vi "实时小时数据单参数上传.vi"(0 "参数数值":T1={"CODMn"=TRUE, "CODCr"=TRUE, "DO"=TRUE, "铜"=TRUE, "PH"=TRUE, "氨氮"=TRUE, "比电导率"=TRUE, "水温"=TRUE, "盐度(海水)"=TRUE, "浊度"=TRUE, "总氮"=TRUE, "总磷"=TRUE, "叶绿素a"=TRUE, "藻密度"=TRUE, "水位"=TRUE, "流速"=TRUE, "瞬时流量"=TRUE, "累积流量"=TRUE}) -> (4 "数据发送起始时间":timestamp format="%<%.3X\n%Y/%m/%d>T", 6 "实时小时数据上传":bool, 15 "error out":errorcluster)   [LabVIEW 2016, in "数据传输系统.lvlib"]
uses:
  <vilib>/Utility/config.llb/Write Key (String).vi
  <vilib>/Utility/config.llb/NI_LVConfig.lvlib
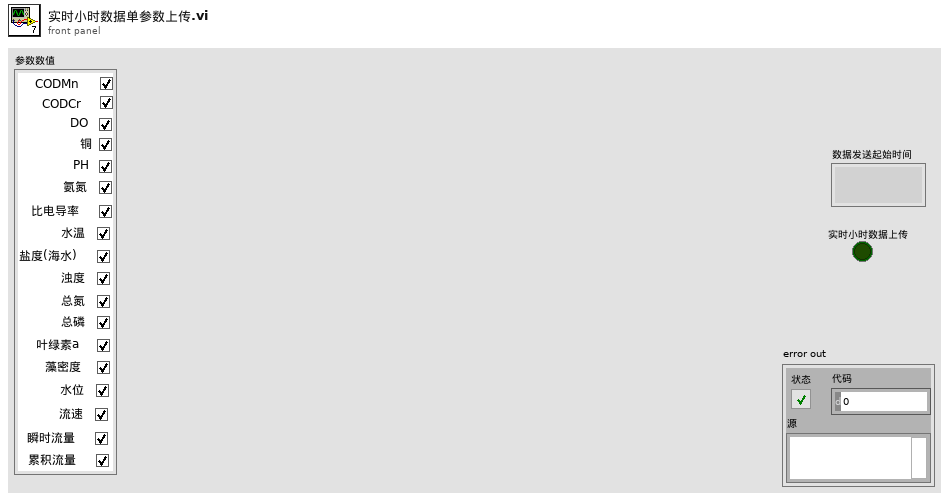
[diagram p1: front panel]
types:
  T1 = cluster{"CODMn":bool, "CODCr":bool, "DO":bool, "铜":bool, "PH":bool, "氨氮":bool, "比电导率":bool, "水温":bool, "盐度(海水)":bool, "浊度":bool, "总氮":bool, "总磷":bool, "叶绿素a":bool, "藻密度":bool, "水位":bool, "流速":bool, "瞬时流量":bool, "累积流量":bool}
  T2 = typedef "NI_LVConfig.lvlib/Config Data RefNum.ctl" = refnum<k1>
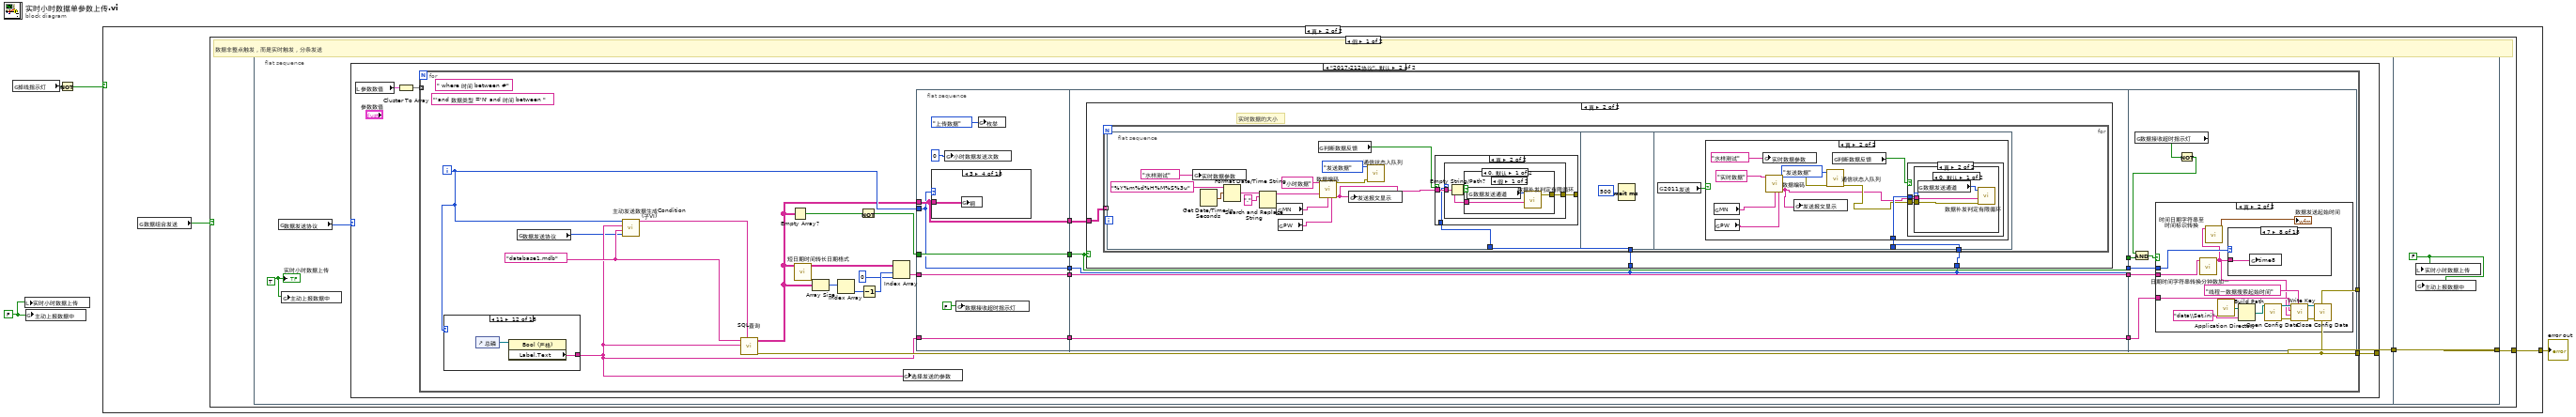
[diagram p0: block diagram]
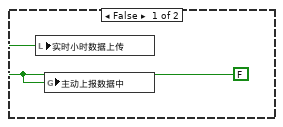
[diagram p2: hidden frame]
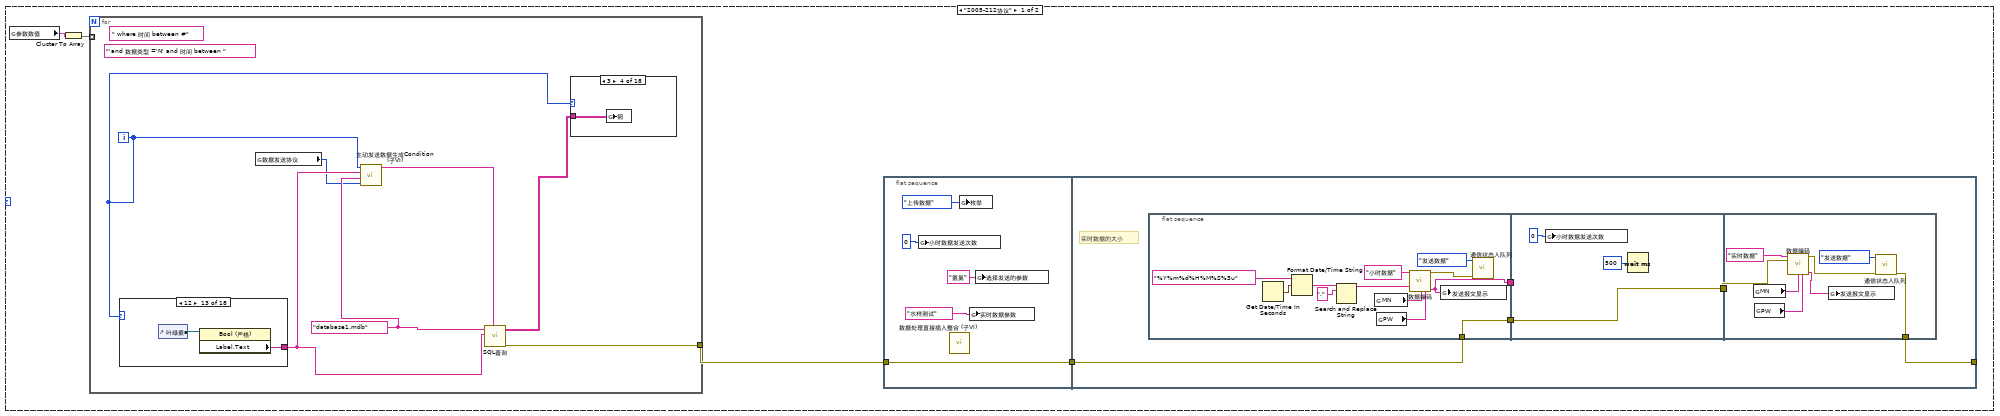
[diagram p3: hidden frame]
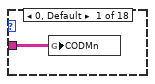
[diagram p4: hidden frame]
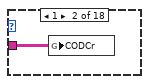
[diagram p5: hidden frame]
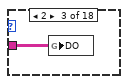
[diagram p6: hidden frame]
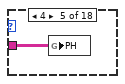
[diagram p7: hidden frame]
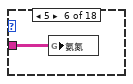
[diagram p8: hidden frame]
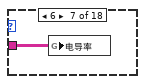
[diagram p9: hidden frame]
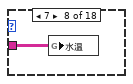
[diagram p10: hidden frame]
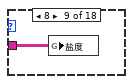
[diagram p11: hidden frame]
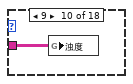
[diagram p12: hidden frame]
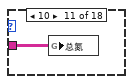
[diagram p13: hidden frame]
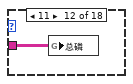
[diagram p14: hidden frame]
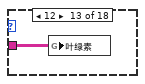
[diagram p15: hidden frame]
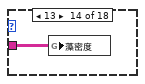
[diagram p16: hidden frame]
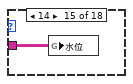
[diagram p17: hidden frame]
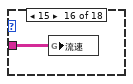
[diagram p18: hidden frame]
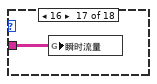
[diagram p19: hidden frame]
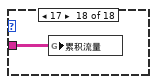
[diagram p20: hidden frame]
diagram:
  w4 = FALSE ("小时数据上传")
  n1 = global read "全局 数据发送重叠.vi" "掉线指示灯"() -> (w3:bool)
  n2 = local write "实时小时数据上传"(w4) -> ()
  n3 = global write "全局 数据发送重叠.vi" "主动上报数据中"(w4) -> ()
  n4 = Not(x=w3) -> (.not. x?=w2:bool)
  n5 = case shown="真" w2 {
    tunnel: [_ w7] -> w1
    frame False {
      w5 = FALSE ("小时数据上传")
      n6 = local write "实时小时数据上传"(w5) -> ()
      n7 = global write "全局 数据发送重叠.vi" "主动上报数据中"(w5) -> ()
    }
    frame True {
      n8 = global read "断电保存全局.vi" "数据组合发送"() -> (w6:bool)
      n9 = case shown="假" w6 {
        tunnel: [w8 _] -> w7
        frame False {
          # "数据非整点触发，而是实时触发，分条发送"
          n10 = flat-sequence {
            tunnel: [w12] -> w9
            tunnel: [w291] -> w8
            tunnel: w9 -> [w291]
            frame #0 {
              w11 = TRUE ("小时数据上传")
              n11 = global read "断电保存全局.vi" "数据发送协议"() -> (w10:enum16{"2005-212协议", "2017-212协议"})
              n12 = global write "全局 数据发送重叠.vi" "主动上报数据中"(w11) -> ()
              n13 = case shown="\"2017-212协议\", 默认" w10 {
                tunnel: [_ w111] -> w12
                frame "2005-212协议" {
                  n14 = global read "全局1.vi" "参数数值"() -> (w13:T1)
                  n15 = Cluster To Array(cluster=w13) -> (array=w16:bool[])
                  n16 = for {
                    tunnel: w16 -> [_] mode=indexing
                    tunnel: [w56] -> w15
                    i -> [w54]
                    (unwired) " where 时间 between #"
                    w52 = "database1.mdb" ("database")
                    (unwired) "'and 数据类型 ='N' and 时间 between "
                    n17 = case shown="12" w54 {
                      tunnel: [w75 w77 w79 w81 w83 w85 w87 w89 w91 w93 w95 w97 w99 w101 w103 w105 w107 w109] -> w53
                      frame 0, Default {
                        n18 = control-ref of="CODMn"() -> (w76:refnum<vi>)
                        n19 = property class="Bool (严格)"(reference=w76) -> ("Label.Text"=w75:string)  [unwired: 1 in, 2 out]
                      }
                      frame 1 {
                        n20 = control-ref of="CODCr"() -> (w78:refnum<vi>)
                        n21 = property class="Bool (严格)"(reference=w78) -> ("Label.Text"=w77:string)  [unwired: 1 in, 2 out]
                      }
                      frame 2 {
                        n22 = control-ref of="DO"() -> (w80:refnum<vi>)
                        n23 = property class="Bool (严格)"(reference=w80) -> ("Label.Text"=w79:string)  [unwired: 1 in, 2 out]
                      }
                      frame 3 {
                        n24 = control-ref of="铜"() -> (w82:refnum<vi>)
                        n25 = property class="Bool (严格)"(reference=w82) -> ("Label.Text"=w81:string)  [unwired: 1 in, 2 out]
                      }
                      frame 4 {
                        n26 = control-ref of="PH"() -> (w84:refnum<vi>)
                        n27 = property class="Bool (严格)"(reference=w84) -> ("Label.Text"=w83:string)  [unwired: 1 in, 2 out]
                      }
                      frame 5 {
                        n28 = control-ref of="氨氮"() -> (w86:refnum<vi>)
                        n29 = property class="Bool (严格)"(reference=w86) -> ("Label.Text"=w85:string)  [unwired: 1 in, 2 out]
                      }
                      frame 6 {
                        n30 = control-ref of="比电导率"() -> (w88:refnum<vi>)
                        n31 = property class="Bool (严格)"(reference=w88) -> ("Label.Text"=w87:string)  [unwired: 1 in, 2 out]
                      }
                      frame 7 {
                        n32 = control-ref of="水温"() -> (w90:refnum<vi>)
                        n33 = property class="Bool (严格)"(reference=w90) -> ("Label.Text"=w89:string)  [unwired: 1 in, 2 out]
                      }
                      frame 8 {
                        n34 = control-ref of="盐度(海水)"() -> (w92:refnum<vi>)
                        n35 = property class="Bool (严格)"(reference=w92) -> ("Label.Text"=w91:string)  [unwired: 1 in, 2 out]
                      }
                      frame 9 {
                        n36 = control-ref of="浊度"() -> (w94:refnum<vi>)
                        n37 = property class="Bool (严格)"(reference=w94) -> ("Label.Text"=w93:string)  [unwired: 1 in, 2 out]
                      }
                      frame 10 {
                        n38 = control-ref of="总氮"() -> (w96:refnum<vi>)
                        n39 = property class="Bool (严格)"(reference=w96) -> ("Label.Text"=w95:string)  [unwired: 1 in, 2 out]
                      }
                      frame 11 {
                        n40 = control-ref of="总磷"() -> (w98:refnum<vi>)
                        n41 = property class="Bool (严格)"(reference=w98) -> ("Label.Text"=w97:string)  [unwired: 1 in, 2 out]
                      }
                      frame 12 {
                        n42 = control-ref of="叶绿素a"() -> (w100:refnum<vi>)
                        n43 = property class="Bool (严格)"(reference=w100) -> ("Label.Text"=w99:string)  [unwired: 1 in, 2 out]
                      }
                      frame 13 {
                        n44 = control-ref of="藻密度"() -> (w102:refnum<vi>)
                        n45 = property class="Bool (严格)"(reference=w102) -> ("Label.Text"=w101:string)  [unwired: 1 in, 2 out]
                      }
                      frame 14 {
                        n46 = control-ref of="水位"() -> (w104:refnum<vi>)
                        n47 = property class="Bool (严格)"(reference=w104) -> ("Label.Text"=w103:string)  [unwired: 1 in, 2 out]
                      }
                      frame 15 {
                        n48 = control-ref of="流速"() -> (w106:refnum<vi>)
                        n49 = property class="Bool (严格)"(reference=w106) -> ("Label.Text"=w105:string)  [unwired: 1 in, 2 out]
                      }
                      frame 16 {
                        n50 = control-ref of="瞬时流量"() -> (w108:refnum<vi>)
                        n51 = property class="Bool (严格)"(reference=w108) -> ("Label.Text"=w107:string)  [unwired: 1 in, 2 out]
                      }
                      frame 17 {
                        n52 = control-ref of="累积流量"() -> (w110:refnum<vi>)
                        n53 = property class="Bool (严格)"(reference=w110) -> ("Label.Text"=w109:string)  [unwired: 1 in, 2 out]
                      }
                    }
                    n54 = global read "断电保存全局.vi" "数据发送协议"() -> (w50:enum16{"2005-212协议", "2017-212协议"})
                    n55 = call "主动发送数据生成Condition(子VI).vi"("数据发送协议"=w50, "database"=w52, "Label.Text"=w53, "数值"=w54) -> ("CONDITION"=w51:string)  [unwired: 7 in]
                    n56 = call "SQL查询.vi"("condition"=w51, "table输入"=w53, "database"=w52) -> ("error out"=w56:errorcluster, "data"=w55:string[][])  [unwired: 7 in]
                    n57 = case shown="3" w54 {
                      tunnel: w55 -> [w57 w58 w59 w60 w61 w62 w63 w64 w65 w66 w67 w68 w69 w70 w71 w72 w73 w74]
                      frame 0, Default {
                        n58 = global write "全局 所有参数.vi" "CODMn"(w57) -> ()
                      }
                      frame 1 {
                        n59 = global write "全局 所有参数.vi" "CODCr"(w58) -> ()
                      }
                      frame 2 {
                        n60 = global write "全局 所有参数.vi" "DO"(w59) -> ()
                      }
                      frame 3 {
                        n61 = global write "全局 所有参数.vi" "铜"(w60) -> ()
                      }
                      frame 4 {
                        n62 = global write "全局 所有参数.vi" "PH"(w61) -> ()
                      }
                      frame 5 {
                        n63 = global write "全局 所有参数.vi" "氨氮"(w62) -> ()
                      }
                      frame 6 {
                        n64 = global write "全局 所有参数.vi" "电导率"(w63) -> ()
                      }
                      frame 7 {
                        n65 = global write "全局 所有参数.vi" "水温"(w64) -> ()
                      }
                      frame 8 {
                        n66 = global write "全局 所有参数.vi" "盐度"(w65) -> ()
                      }
                      frame 9 {
                        n67 = global write "全局 所有参数.vi" "浊度"(w66) -> ()
                      }
                      frame 10 {
                        n68 = global write "全局 所有参数.vi" "总氮"(w67) -> ()
                      }
                      frame 11 {
                        n69 = global write "全局 所有参数.vi" "总磷"(w68) -> ()
                      }
                      frame 12 {
                        n70 = global write "全局 所有参数.vi" "叶绿素"(w69) -> ()
                      }
                      frame 13 {
                        n71 = global write "全局 所有参数.vi" "藻密度"(w70) -> ()
                      }
                      frame 14 {
                        n72 = global write "全局 所有参数.vi" "水位"(w71) -> ()
                      }
                      frame 15 {
                        n73 = global write "全局 所有参数.vi" "流速"(w72) -> ()
                      }
                      frame 16 {
                        n74 = global write "全局 所有参数.vi" "瞬时流量"(w73) -> ()
                      }
                      frame 17 {
                        n75 = global write "全局 所有参数.vi" "累积流量"(w74) -> ()
                      }
                    }
                  }
                  n76 = flat-sequence {
                    tunnel: w15 -> [w17]
                    tunnel: [w17] -> w14
                    tunnel: w14 -> [w23]
                    tunnel: [w22] -> _
                    frame #0 {
                      n77 = global write "全局 小时数据发送次数.vi" "小时数据发送次数"(0 ("小时数据发送次数")) -> ()
                      n78 = call "数据处理直接插入整合 (子VI).vi"() -> ()  [unwired: 12 in]
                      n79 = global write "全局1.vi" "枚举"(enum16{"返回请求应答", "上传数据", "返回执行结果"}."上传数据" ("枚举")) -> ()
                      n80 = global write "全局 实时数据参数.vi" "实时数据参数"("水样测试" ("实时数据参数")) -> ()
                      n81 = global write "全局 水样时间.vi" "选择发送的参数"("氨氮" ("选择发送的参数")) -> ()
                    }
                    frame #1 {
                      # "实时数据的大小"
                      n82 = flat-sequence {
                        tunnel: [w32] -> w26
                        tunnel: [w27] -> w24
                        tunnel: w23 -> [w27]
                        tunnel: w26 -> [_]
                        tunnel: [w40] -> w25
                        tunnel: w24 -> [w40]
                        tunnel: w25 -> [w48]
                        tunnel: [w42] -> w22
                        frame #0 {
                          n83 = Get Date/Time In Seconds() -> (seconds since 1Jan1904=w35:timestamp)
                          n84 = Format Date/Time String(time format string (%c)="%Y%m%d%H%M%S%3u" ("时间格式字符串(%c)"), seconds (now)=w35) -> (date/time string=w36:string)  [unwired: 1 in]
                          n85 = Search and Replace String(input string=w36, search string="." ("搜索字符串")) -> (result string=w38:string)  [unwired: 6 in, 3 out]
                          n86 = global read "断电保存全局.vi" "MN"() -> (w30:string)
                          n87 = global read "断电保存全局.vi" "PW"() -> (w29:string)
                          n88 = call "数据编码.vi"("table输入"="小时数据" ("新元素/子数组"), "QN"=w38, "MN"=w30, "PW"=w29) -> ("错误常量"=w28:errorcluster, "通讯包字符串"=w32:string)  [unwired: 10 in]
                          n89 = global write "全局1.vi" "发送报文显示"(w32) -> ()
                          n90 = call "通信状态入队列.vi"("错误输入（无错误）"=w28, "枚举"=enum16{"打开连接", "发送数据", "读取数据", "数据处理", "关闭连接"}."发送数据") -> ()  [unwired: 9 in, 1 out]
                        }
                        frame #1 {
                          n91 = global write "全局 小时数据发送次数.vi" "小时数据发送次数"(0 ("小时数据发送次数")) -> ()
                          n92 = Wait (ms)(milliseconds to wait=u32 500 ("等待时间（毫秒）")) -> ()  [unwired: 1 out]
                        }
                        frame #2 {
                          n93 = global read "断电保存全局.vi" "MN"() -> (w44:string)
                          n94 = global read "断电保存全局.vi" "PW"() -> (w45:string)
                          n95 = call "数据编码.vi"("table输入"="实时数据" ("新元素/子数组"), "错误常量 2"=w48, "MN"=w44, "PW"=w45) -> ("错误常量"=w43:errorcluster, "通讯包字符串"=w47:string)  [unwired: 10 in]
                          n96 = global write "全局1.vi" "发送报文显示"(w47) -> ()
                          n97 = call "通信状态入队列.vi"("错误输入（无错误）"=w43, "枚举"=enum16{"打开连接", "发送数据", "读取数据", "数据处理", "关闭连接"}."发送数据") -> ("错误输出"=w42:errorcluster)  [unwired: 9 in]
                        }
                      }
                    }
                  }
                }
                frame "2017-212协议", Default {
                  n98 = local read "参数数值"() -> (w113:T1)
                  n99 = Cluster To Array(cluster=w113) -> (array=w112:bool[])
                  n100 = for {
                    tunnel: w112 -> [_] mode=indexing
                    tunnel: [w123] -> w111
                    tunnel: [w123] -> _
                    i -> [w122]
                    (unwired) " where 时间 between #"
                    w121 = "database1.mdb" ("database")
                    (unwired) "'and 数据类型 ='N' and 时间 between "
                    n101 = case shown="11" w122 {
                      tunnel: [w254 w256 w258 w260 w262 w264 w266 w268 w270 w272 w274 w276 w278 w280 w282 w284 w286 w288] -> w120
                      frame 0, Default {
                        n102 = control-ref of="CODMn"() -> (w255:refnum<vi>)
                        n103 = property class="Bool (严格)"(reference=w255) -> ("Label.Text"=w254:string)  [unwired: 1 in, 2 out]
                      }
                      frame 1 {
                        n104 = control-ref of="CODCr"() -> (w257:refnum<vi>)
                        n105 = property class="Bool (严格)"(reference=w257) -> ("Label.Text"=w256:string)  [unwired: 1 in, 2 out]
                      }
                      frame 2 {
                        n106 = control-ref of="DO"() -> (w259:refnum<vi>)
                        n107 = property class="Bool (严格)"(reference=w259) -> ("Label.Text"=w258:string)  [unwired: 1 in, 2 out]
                      }
                      frame 3 {
                        n108 = control-ref of="铜"() -> (w261:refnum<vi>)
                        n109 = property class="Bool (严格)"(reference=w261) -> ("Label.Text"=w260:string)  [unwired: 1 in, 2 out]
                      }
                      frame 4 {
                        n110 = control-ref of="PH"() -> (w263:refnum<vi>)
                        n111 = property class="Bool (严格)"(reference=w263) -> ("Label.Text"=w262:string)  [unwired: 1 in, 2 out]
                      }
                      frame 5 {
                        n112 = control-ref of="氨氮"() -> (w265:refnum<vi>)
                        n113 = property class="Bool (严格)"(reference=w265) -> ("Label.Text"=w264:string)  [unwired: 1 in, 2 out]
                      }
                      frame 6 {
                        n114 = control-ref of="比电导率"() -> (w267:refnum<vi>)
                        n115 = property class="Bool (严格)"(reference=w267) -> ("Label.Text"=w266:string)  [unwired: 1 in, 2 out]
                      }
                      frame 7 {
                        n116 = control-ref of="水温"() -> (w269:refnum<vi>)
                        n117 = property class="Bool (严格)"(reference=w269) -> ("Label.Text"=w268:string)  [unwired: 1 in, 2 out]
                      }
                      frame 8 {
                        n118 = control-ref of="盐度(海水)"() -> (w271:refnum<vi>)
                        n119 = property class="Bool (严格)"(reference=w271) -> ("Label.Text"=w270:string)  [unwired: 1 in, 2 out]
                      }
                      frame 9 {
                        n120 = control-ref of="浊度"() -> (w273:refnum<vi>)
                        n121 = property class="Bool (严格)"(reference=w273) -> ("Label.Text"=w272:string)  [unwired: 1 in, 2 out]
                      }
                      frame 10 {
                        n122 = control-ref of="总氮"() -> (w275:refnum<vi>)
                        n123 = property class="Bool (严格)"(reference=w275) -> ("Label.Text"=w274:string)  [unwired: 1 in, 2 out]
                      }
                      frame 11 {
                        n124 = control-ref of="总磷"() -> (w277:refnum<vi>)
                        n125 = property class="Bool (严格)"(reference=w277) -> ("Label.Text"=w276:string)  [unwired: 1 in, 2 out]
                      }
                      frame 12 {
                        n126 = control-ref of="叶绿素a"() -> (w279:refnum<vi>)
                        n127 = property class="Bool (严格)"(reference=w279) -> ("Label.Text"=w278:string)  [unwired: 1 in, 2 out]
                      }
                      frame 13 {
                        n128 = control-ref of="藻密度"() -> (w281:refnum<vi>)
                        n129 = property class="Bool (严格)"(reference=w281) -> ("Label.Text"=w280:string)  [unwired: 1 in, 2 out]
                      }
                      frame 14 {
                        n130 = control-ref of="水位"() -> (w283:refnum<vi>)
                        n131 = property class="Bool (严格)"(reference=w283) -> ("Label.Text"=w282:string)  [unwired: 1 in, 2 out]
                      }
                      frame 15 {
                        n132 = control-ref of="流速"() -> (w285:refnum<vi>)
                        n133 = property class="Bool (严格)"(reference=w285) -> ("Label.Text"=w284:string)  [unwired: 1 in, 2 out]
                      }
                      frame 16 {
                        n134 = control-ref of="瞬时流量"() -> (w287:refnum<vi>)
                        n135 = property class="Bool (严格)"(reference=w287) -> ("Label.Text"=w286:string)  [unwired: 1 in, 2 out]
                      }
                      frame 17 {
                        n136 = control-ref of="累积流量"() -> (w289:refnum<vi>)
                        n137 = property class="Bool (严格)"(reference=w289) -> ("Label.Text"=w288:string)  [unwired: 1 in, 2 out]
                      }
                    }
                    n138 = global read "断电保存全局.vi" "数据发送协议"() -> (w119:enum16{"2005-212协议", "2017-212协议"})
                    n139 = call "主动发送数据生成Condition(子VI).vi"("数据发送协议"=w119, "database"=w121, "Label.Text"=w120, "数值"=w122) -> ("CONDITION"=w137:string)  [unwired: 7 in]
                    n140 = call "SQL查询.vi"("condition"=w137, "table输入"=w120, "database"=w121) -> ("error out"=w123:errorcluster, "data"=w116:string[][])  [unwired: 7 in]
                    n141 = Empty Array?(array=w116) -> (empty?=w136:bool)
                    n142 = call "短日期时间转长日期格式.vi"("data"=w116) -> ("输出数组"=w135:string[][])  [unwired: 10 in]
                    n143 = Array Size(array=w116) -> (size(s)=w118:i32[])
                    n144 = Index Array(array=w118) -> (element=w117:i32)  [unwired: 1 in]
                    n145 = Not(x=w136) -> (.not. x?=w132:bool)
                    n146 = Decrement(x=w117) -> (x-1=w115:i32)
                    n147 = Index Array(array=w135, index (row)=w115, index (col)=0 ("禁用的索引 (列)")) -> (element=w129:string)
                    n148 = global write "全局 水样时间.vi" "选择发送的参数"(w120) -> ()
                    n149 = flat-sequence {
                      tunnel: [w145] -> w134
                      tunnel: [w144] -> w133
                      tunnel: w132 -> [w145]
                      tunnel: w116 -> [w144]
                      tunnel: w122 -> [w139]
                      tunnel: w120 -> [w141]
                      tunnel: [w141] -> w130
                      tunnel: w129 -> [w140]
                      tunnel: [w140] -> w127
                      tunnel: [w139] -> w124
                      tunnel: w134 -> [w165]
                      tunnel: w133 -> [w168]
                      tunnel: [w167] -> w131
                      tunnel: w130 -> [w167]
                      tunnel: [w166] -> w128
                      tunnel: w127 -> [w166]
                      tunnel: [w165] -> w126
                      tunnel: [w164] -> w125
                      tunnel: w124 -> [w164]
                      tunnel: w131 -> [w222]
                      tunnel: w128 -> [w221]
                      tunnel: w126 -> [w219]
                      tunnel: w125 -> [w220]
                      frame #0 {
                        n150 = case shown="3" w139 {
                          tunnel: w144 -> [w146 w147 w148 w149 w150 w151 w152 w153 w154 w155 w156 w157 w158 w159 w160 w161 w162 w163]
                          frame 0, Default {
                            n151 = global write "全局 所有参数.vi" "CODMn"(w146) -> ()
                          }
                          frame 1 {
                            n152 = global write "全局 所有参数.vi" "CODCr"(w147) -> ()
                          }
                          frame 2 {
                            n153 = global write "全局 所有参数.vi" "DO"(w148) -> ()
                          }
                          frame 3 {
                            n154 = global write "全局 所有参数.vi" "铜"(w149) -> ()
                          }
                          frame 4 {
                            n155 = global write "全局 所有参数.vi" "PH"(w150) -> ()
                          }
                          frame 5 {
                            n156 = global write "全局 所有参数.vi" "氨氮"(w151) -> ()
                          }
                          frame 6 {
                            n157 = global write "全局 所有参数.vi" "电导率"(w152) -> ()
                          }
                          frame 7 {
                            n158 = global write "全局 所有参数.vi" "水温"(w153) -> ()
                          }
                          frame 8 {
                            n159 = global write "全局 所有参数.vi" "盐度"(w154) -> ()
                          }
                          frame 9 {
                            n160 = global write "全局 所有参数.vi" "浊度"(w155) -> ()
                          }
                          frame 10 {
                            n161 = global write "全局 所有参数.vi" "总氮"(w156) -> ()
                          }
                          frame 11 {
                            n162 = global write "全局 所有参数.vi" "总磷"(w157) -> ()
                          }
                          frame 12 {
                            n163 = global write "全局 所有参数.vi" "叶绿素"(w158) -> ()
                          }
                          frame 13 {
                            n164 = global write "全局 所有参数.vi" "藻密度"(w159) -> ()
                          }
                          frame 14 {
                            n165 = global write "全局 所有参数.vi" "水位"(w160) -> ()
                          }
                          frame 15 {
                            n166 = global write "全局 所有参数.vi" "流速"(w161) -> ()
                          }
                          frame 16 {
                            n167 = global write "全局 所有参数.vi" "瞬时流量"(w162) -> ()
                          }
                          frame 17 {
                            n168 = global write "全局 所有参数.vi" "累积流量"(w163) -> ()
                          }
                        }
                        n169 = global write "全局 小时数据发送次数.vi" "小时数据发送次数"(0 ("小时数据发送次数")) -> ()
                        n170 = global write "全局 数据发送重叠.vi" "数据接收超时指示灯"(FALSE ("数据接收超时指示灯")) -> ()
                        n171 = global write "全局1.vi" "枚举"(enum16{"返回请求应答", "上传数据", "返回执行结果"}."上传数据" ("枚举")) -> ()
                      }
                      frame #1 {
                        n172 = case shown="真" w165 {
                          tunnel: w168 -> [_ w171]
                          tunnel: w164 -> [_ w170]
                          tunnel: w164 -> [_ w169]
                          frame False {
                          }
                          frame True {
                            # "实时数据的大小"
                            n173 = for {
                              tunnel: w171 -> [_] mode=indexing
                              tunnel: w170 -> [w173]
                              tunnel: w169 -> [w172]
                              n174 = flat-sequence {
                                tunnel: w173 -> [w187]
                                tunnel: w172 -> [w198]
                                frame #0 {
                                n175 = global write "全局 实时数据参数.vi" "实时数据参数"("水样测试" ("实时数据参数")) -> ()
                                n176 = Get Date/Time In Seconds() -> (seconds since 1Jan1904=w183:timestamp)
                                n177 = Format Date/Time String(time format string (%c)="%Y%m%d%H%M%S%3u" ("时间格式字符串(%c)"), seconds (now)=w183) -> (date/time string=w184:string)  [unwired: 1 in]
                                n178 = Search and Replace String(input string=w184, search string="." ("搜索字符串")) -> (result string=w186:string)  [unwired: 6 in, 3 out]
                                n179 = global read "断电保存全局.vi" "MN"() -> (w179:string)
                                n180 = global read "断电保存全局.vi" "PW"() -> (w178:string)
                                n181 = global read "断电保存全局.vi" "判断数据反馈"() -> (w175:bool)
                                n182 = call "数据编码.vi"("table输入"="小时数据" ("新元素/子数组"), "QN"=w186, "MN"=w179, "PW"=w178) -> ("错误常量"=w176:errorcluster, "通讯包字符串"=w174:string)  [unwired: 10 in]
                                n183 = global write "全局1.vi" "发送报文显示"(w174) -> ()
                                n184 = call "通信状态入队列.vi"("错误输入（无错误）"=w176, "枚举"=enum16{"打开连接", "发送数据", "读取数据", "数据处理", "关闭连接"}."发送数据") -> ()  [unwired: 9 in, 1 out]
                                n185 = case shown="真" w175 {
                                tunnel: [_ w190] -> _
                                tunnel: w174 -> [_ w189]
                                tunnel: w187 -> [_ w188]
                                frame False {
                                }
                                frame True {
                                n186 = case shown="0, 默认" w188 {
                                tunnel: [w192 _] -> w190
                                tunnel: w189 -> [w191 _]
                                frame 0, Default {
                                n187 = Empty String/Path?(string/path=w191) -> (empty?=w193:bool)
                                n188 = case shown="假" w193 {
                                tunnel: [w196 _] -> w192
                                tunnel: w191 -> [w195 _]
                                frame False {
                                n189 = global read "断电保存全局.vi" "数据发送通道"() -> (w194:enum16{"TCP", "VISA"})
                                n190 = call "数据补发判定有限循环.vi"("数据输入"=w195, "数据发送通道"=w194) -> ("error out"=w196:errorcluster)  [unwired: 9 in]
                                }
                                frame True {
                                }
                                }
                                }
                                frame 14..17 {
                                }
                                }
                                }
                                }
                                }
                                frame #1 {
                                n191 = Wait (ms)(milliseconds to wait=u32 500 ("等待时间（毫秒）")) -> ()  [unwired: 1 out]
                                }
                                frame #2 {
                                n192 = global read "断电保存全局.vi" "2011发送"() -> (w199:bool)
                                n193 = case shown="真" w199 {
                                tunnel: w198 -> [_ w209]
                                frame False {
                                }
                                frame True {
                                n194 = global read "断电保存全局.vi" "MN"() -> (w204:string)
                                n195 = global read "断电保存全局.vi" "PW"() -> (w203:string)
                                n196 = global write "全局 实时数据参数.vi" "实时数据参数"("水样测试" ("实时数据参数")) -> ()
                                n197 = call "数据编码.vi"("table输入"="实时数据" ("新元素/子数组"), "MN"=w204, "PW"=w203) -> ("错误常量"=w205:errorcluster, "通讯包字符串"=w200:string)  [unwired: 11 in]
                                n198 = global write "全局1.vi" "发送报文显示"(w200) -> ()
                                n199 = call "通信状态入队列.vi"("错误输入（无错误）"=w205, "枚举"=enum16{"打开连接", "发送数据", "读取数据", "数据处理", "关闭连接"}."发送数据") -> ("错误输出"=w202:errorcluster)  [unwired: 9 in]
                                n200 = global read "断电保存全局.vi" "判断数据反馈"() -> (w201:bool)
                                n201 = case shown="真" w201 {
                                tunnel: w200 -> [_ w212]
                                tunnel: w202 -> [_ w211]
                                tunnel: w209 -> [_ w210]
                                frame False {
                                }
                                frame True {
                                n202 = case shown="0, 默认" w210 {
                                tunnel: w212 -> [w215 _]
                                tunnel: w211 -> [w214 _]
                                frame 0, Default {
                                n203 = global read "断电保存全局.vi" "数据发送通道"() -> (w213:enum16{"TCP", "VISA"})
                                n204 = call "数据补发判定有限循环.vi"("错误输入（无错误）"=w214, "数据输入"=w215, "数据发送通道"=w213) -> ()  [unwired: 8 in, 1 out]
                                }
                                frame 14..17 {
                                }
                                }
                                }
                                }
                                }
                                }
                                }
                              }
                            }
                          }
                        }
                      }
                      frame #2 {
                        n205 = global read "全局 数据发送重叠.vi" "数据接收超时指示灯"() -> (w216:bool)
                        n206 = Not(x=w216) -> (.not. x?=w217:bool)
                        n207 = Compound Arithmetic op=AND ("复合运算")(w217, w219) -> (w218:bool)
                        n208 = case shown="真" w218 {
                          tunnel: w221 -> [_ w225]
                          tunnel: w220 -> [_ w235]
                          tunnel: w222 -> [_ w226]
                          frame False {
                          }
                          frame True {
                            n209 = call "日期时间字符串转换分钟数加一.vi"("data[0]"=w225) -> ("日期/时间字符串"=w224:string)  [unwired: 10 in]
                            n210 = call "时间日期字符串至时间标识转换.vi"("时间日期字符串"=w224) -> ("时间标识"=→"数据发送起始时间":timestamp)  [unwired: 10 in]
                            n211 = call <vilib>:"Application Directory.vi"() -> ("Application Directory"=w227:path)
                            n212 = case shown="7" w235 {
                              tunnel: w224 -> [w236 w237 w238 w239 w240 w241 w242 w243 w244 w245 w246 w247 w248 w249 w250 w251 w252 w253]
                              frame 0, Default {
                                n213 = global write "全局 水样时间.vi" "time1"(w236) -> ()
                              }
                              frame 1 {
                                n214 = global write "全局 水样时间.vi" "time2"(w237) -> ()
                              }
                              frame 2 {
                                n215 = global write "全局 水样时间.vi" "time3"(w238) -> ()
                              }
                              frame 3 {
                                n216 = global write "全局 水样时间.vi" "time4"(w239) -> ()
                              }
                              frame 4 {
                                n217 = global write "全局 水样时间.vi" "time5"(w240) -> ()
                              }
                              frame 5 {
                                n218 = global write "全局 水样时间.vi" "time6"(w241) -> ()
                              }
                              frame 6 {
                                n219 = global write "全局 水样时间.vi" "time7"(w242) -> ()
                              }
                              frame 7 {
                                n220 = global write "全局 水样时间.vi" "time8"(w243) -> ()
                              }
                              frame 8 {
                                n221 = global write "全局 水样时间.vi" "time9"(w244) -> ()
                              }
                              frame 9 {
                                n222 = global write "全局 水样时间.vi" "time10"(w245) -> ()
                              }
                              frame 10 {
                                n223 = global write "全局 水样时间.vi" "time11"(w246) -> ()
                              }
                              frame 11 {
                                n224 = global write "全局 水样时间.vi" "time12"(w247) -> ()
                              }
                              frame 12 {
                                n225 = global write "全局 水样时间.vi" "time13"(w248) -> ()
                              }
                              frame 13 {
                                n226 = global write "全局 水样时间.vi" "time14"(w249) -> ()
                              }
                              frame 14 {
                                n227 = global write "全局 水样时间.vi" "time15"(w250) -> ()
                              }
                              frame 15 {
                                n228 = global write "全局 水样时间.vi" "time16"(w251) -> ()
                              }
                              frame 16 {
                                n229 = global write "全局 水样时间.vi" "time17"(w252) -> ()
                              }
                              frame 17 {
                                n230 = global write "全局 水样时间.vi" "time18"(w253) -> ()
                              }
                            }
                            n231 = Build Path(base path=w227, name or relative path="data\\Set.ini" ("名称或相对路径")) -> (appended path=w229:path)
                            n232 = call <vilib>:"Open Config Data.vi"("configuration file path"=w229) -> ("error out"=w231:errorcluster, "refnum"=w230:T2)  [unwired: 8 in, 1 out]
                            n233 = call-poly <vilib>:"Write Key.vi"("section"="线程一数据搜索起始时间", "error in (no error)"=w231, "value"=w224, "key"=w226, "refnum"=w230) -> ("error out"=w233:errorcluster, "refnum out"=w232:T2)  [unwired: 4 in, 1 out]
                            n234 = call <vilib>:"Close Config Data.vi"("error in (no error)"=w233, "refnum"=w232) -> ()  [unwired: 8 in, 2 out]
                          }
                        }
                      }
                    }
                  }
                }
              }
              "实时小时数据上传" <- w11
            }
            frame #1 {
              w290 = FALSE ("小时数据上传")
              n235 = local write "实时小时数据上传"(w290) -> ()
              n236 = global write "全局 数据发送重叠.vi" "主动上报数据中"(w290) -> ()
            }
          }
        }
        frame True {
          # "数据整点触发，整条发送"
        }
      }
    }
  }
  "error out" <- w1
